vi "Holodrive.vi"(0 "Translation X":dbl, 5 "Translation Y":dbl, 7 "Angular":dbl, 9 "Robot Length":dbl=22.0, 11 "Robot Width":dbl=20.5) -> (2 "FL Rot":dbl, 3 "FR Rot":dbl, 4 "BL Rot":dbl, 6 "BR Rot":dbl, 10 "BR Drive":dbl, 13 "FL Drive":dbl, 14 "FR Drive":dbl, 15 "BL Drive":dbl)   [LabVIEW 2014]
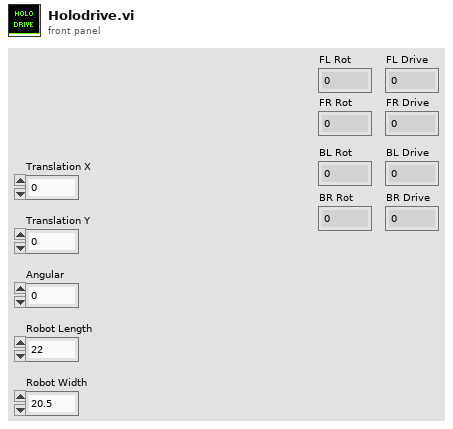
[diagram p1: front panel]
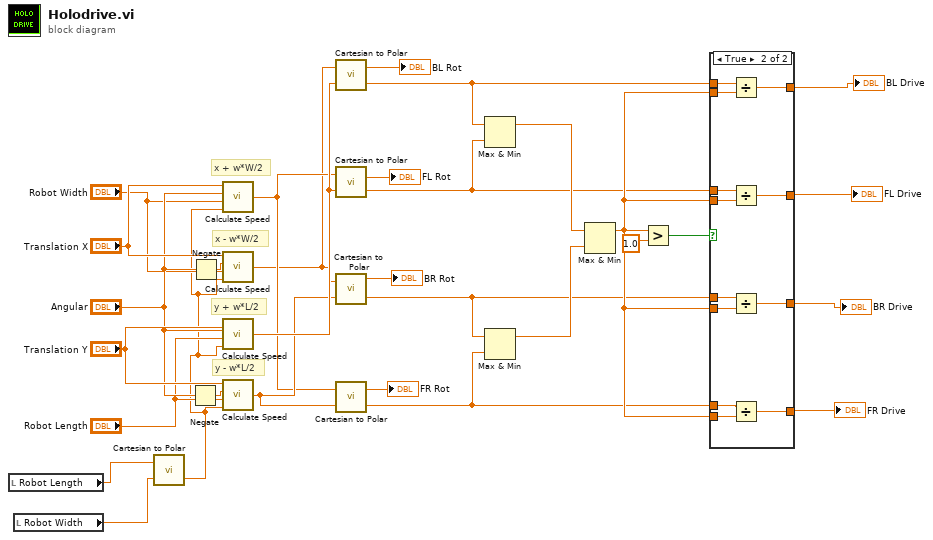
[diagram p0: block diagram]
diagram:
  # "y - w*L/2"
  # "y + w*L/2"
  # "x - w*W/2"
  # "x + w*W/2"
  n1 = local read "Robot Length"() -> (w7:dbl)
  n2 = local read "Robot Width"() -> (w6:dbl)
  n3 = call "Cartesian to Polar.vi"("y"=w6, "x"=w7) -> ("magnitude"=w5:dbl)  [unwired: 1 out]
  n4 = Negate(x="Angular") -> (-x=w29:dbl)
  n5 = Negate(x="Angular") -> (-x=w28:dbl)
  n6 = call "Calculate Speed.vi"("radius"=w5, "dimension"="Robot Width", "rotational"="Angular", "translational"="Translation X") -> ("speed"=w2:dbl)
  n7 = call "Calculate Speed.vi"("radius"=w5, "dimension"="Robot Width", "rotational"=w28, "translational"="Translation X") -> ("speed"=w1:dbl)
  n8 = call "Calculate Speed.vi"("radius"=w5, "dimension"="Robot Length", "rotational"="Angular", "translational"="Translation Y") -> ("speed"=w4:dbl)
  n9 = call "Calculate Speed.vi"("radius"=w5, "dimension"="Robot Length", "rotational"=w29, "translational"="Translation Y") -> ("speed"=w3:dbl)
  n10 = call "Cartesian to Polar.vi"("y"=w4, "x"=w1) -> ("magnitude"=w19:dbl, "angle"=→"BL Rot":dbl)
  n11 = call "Cartesian to Polar.vi"("y"=w4, "x"=w2) -> ("magnitude"=w18:dbl, "angle"=→"FL Rot":dbl)
  n12 = call "Cartesian to Polar.vi"("y"=w3, "x"=w1) -> ("magnitude"=w17:dbl, "angle"=→"BR Rot":dbl)
  n13 = call "Cartesian to Polar.vi"("y"=w3, "x"=w2) -> ("magnitude"=w16:dbl, "angle"=→"FR Rot":dbl)
  n14 = Max & Min(x=w19, y=w18) -> (max(x,y)=w24:dbl)  [unwired: 1 out]
  n15 = Max & Min(x=w17, y=w16) -> (max(x,y)=w23:dbl)  [unwired: 1 out]
  n16 = Max & Min(x=w24, y=w23) -> (max(x,y)=w20:dbl)  [unwired: 1 out]
  n17 = Greater?(x=w20, y=1.0) -> (0:w21:bool)
  n18 = case shown="True" w21 {
    tunnel: w20 -> [_ w47]
    tunnel: w20 -> [_ w46]
    tunnel: w20 -> [_ w45]
    tunnel: w20 -> [_ w44]
    tunnel: [w35 w43] -> w11
    tunnel: [w34 w42] -> w10
    tunnel: [w33 w41] -> w9
    tunnel: [w32 w40] -> w8
    tunnel: w19 -> [w35 w39]
    tunnel: w18 -> [w34 w38]
    tunnel: w17 -> [w33 w37]
    tunnel: w16 -> [w32 w36]
    frame False {
    }
    frame True {
      n19 = Divide(x=w39, y=w44) -> (x/y=w43:dbl)
      n20 = Divide(x=w38, y=w45) -> (x/y=w42:dbl)
      n21 = Divide(x=w37, y=w46) -> (x/y=w41:dbl)
      n22 = Divide(x=w36, y=w47) -> (x/y=w40:dbl)
    }
  }
  "FL Drive" <- w10
  "FR Drive" <- w8
  "BL Drive" <- w11
  "BR Drive" <- w9
